vi "Get Sections.vi"(8 "error in (no error)":errorcluster, 11 "Configuration Reference In":refnum<data-value>) -> (0 "error out":errorcluster, 2 "Section names":string[](array[string]), 3 "Configuration Reference Out":refnum<data-value>)   [LabVIEW 2012, in "configlib.lvlib"]
uses:
  configlib.lvlib
  Configuration File Definition.ctl
  File Options.ctl
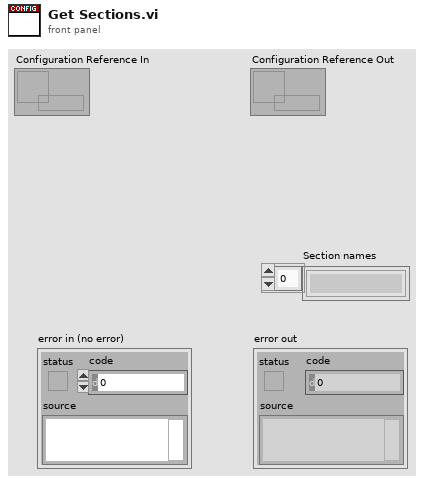
[diagram p1: front panel]
types:
  T1 = typedef "configlib.lvlib/Configuration File Definition.ctl" = cluster{"dirty":bool, "path":path, "Fileopts":T2, "Section Lookup":variant, "Key Lookup":variant, "Raw File":string[]}
  T2 = typedef "configlib.lvlib/File Options.ctl" = cluster{"Name/Value delimiter (\"=\")":string, "Comment delimiter (\";\")":string}
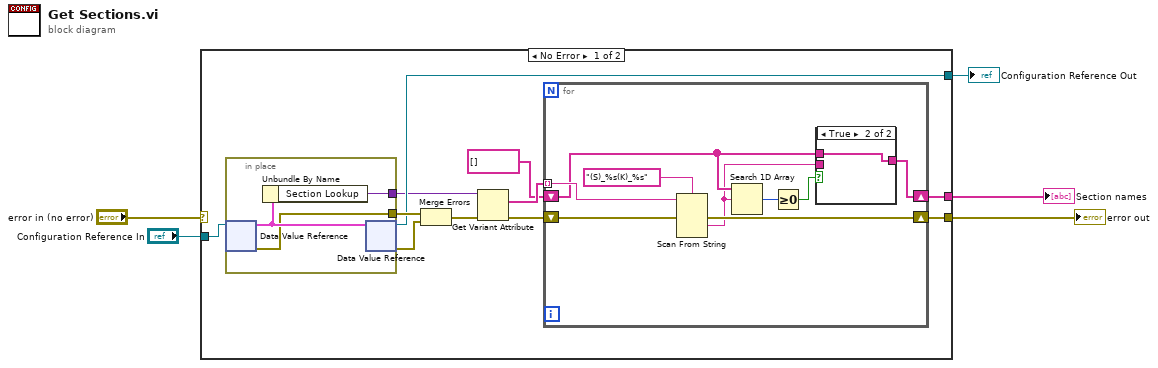
[diagram p0: block diagram]
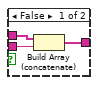
[diagram p2: hidden frame]
diagram:
  n1 = case shown="No Error" "error in (no error)" {
    selector: "error in (no error)" -> [_ w34]
    tunnel: [w8 w34] -> w4
    tunnel: "Configuration Reference In" -> [w16 w33]
    tunnel: [w13 w33] -> w2
    tunnel: [w6 _] -> w1
    frame No Error {
      n2 = in-place {
        in-place-border: [w31] -> w11
        in-place-border: [w30] -> w15
        n3 = in-place-dvr #1(w16) -> (w32:T1, w30:errorcluster)
        n4 = Unbundle By Name(w32) -> ("Section Lookup"=w31:variant)
        n5 = in-place-dvr #1(w32) -> (w13:refnum<data-value>, w14:errorcluster)
      }
      n6 = Merge Errors(w15, w14) -> (w12:errorcluster)
      n7 = Get Variant Attribute(Variant=w11, error in=w12) -> (names=w10:string[], error out=w9:errorcluster)  [unwired: 2 in, 2 out]
      n8 = for {
        tunnel: w10 -> [w23] mode=indexing
        shift-right: [w24] -> w8
        shift-left: w9 -> [w25]
        shift-right: [w17] -> w6
        shift-left: string[] [] -> [w19]
        n9 = Scan From String(format string="(S)_%s(K)_%s", input string=w23, error in=w25) -> (error out=w24:errorcluster, output 1=w18:string)  [unwired: 4 in, 2 out]
        n10 = Search 1D Array(1D array=w19, element=w18) -> (index of element=w21:i32)  [unwired: 1 in]
        n11 = Greater Or Equal To 0?(x=w21) -> (x >= 0?=w20:bool)
        n12 = case shown="True" w20 {
          tunnel: w19 -> [w28 w29]
          tunnel: w18 -> [w27 _]
          tunnel: [w26 w29] -> w17
          frame False {
            n13 = Build Array (concatenate)(w28, w27) -> (w26:string[])
          }
          frame True {
          }
        }
      }
    }
    frame Error {
    }
  }
  "Configuration Reference Out" <- w2
  "error out" <- w4
  "Section names" <- w1
